vi "2021_day3_task2.vi"() -> ()   [LabVIEW 2021]
panel:
  out "life support rating":i32
  out "CO2 scrubber rating":i32
  out "oxygen generator rating":i32
  out "power consumption":u32
  out "Epsilon (DEC)":u32
  out "Gamma (DEC)":u32
  out "GAMA":bool[](array[boolean])
  out "EPSILON":bool[](array[boolean])
  out "size(s)":i32
  out "Array 2":i32[](array[numeric])
  out "Array":i32[][](array[numeric])
  out "array 2":string[](array[string])
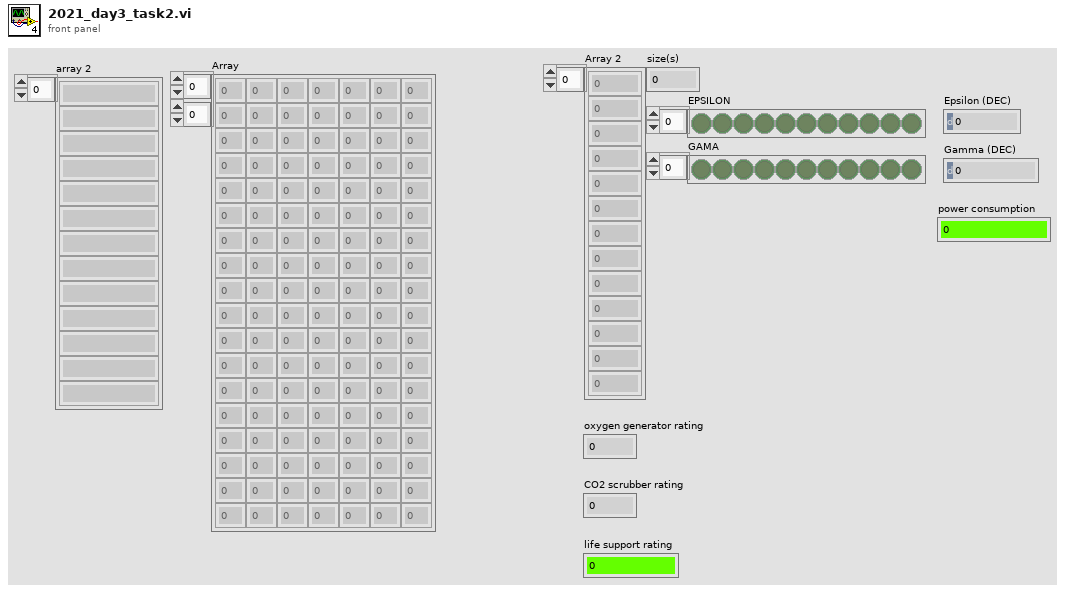
[diagram p1: front panel]
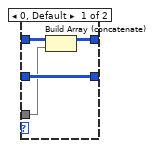
[diagram p2: hidden frame]
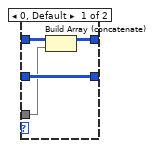
[diagram p3: hidden frame]
diagram:
  (unwired) "00100\n11110\n10110\n10111\n10101\n01111\n00111\n11100\n10000\n11001\n00010\n01010"
  n1 = Spreadsheet String To Array(delimiter (Tab)="\n", format string="%s", spreadsheet string="000111111001\n111011110110\n101111111000\n111100100110\n001111011000\n011100010110\n000101001001\n100001100101\n000011111100\n110000101000\n011110110101\n011000111100\n011000001011\n010111101101\n011111100010\n100110001111\n100111100100\n111110010100\n101001001110\n110101111110\n110110100000\n001010001110\n101100001100\n111001011000\n100101111111\n001001010100\n100111011000\n100101100000\n010001010101\n000111001100\n001100011110\n101100010101\n111011000011\n010000001110\n110000000110\n001010110000\n100011001111\n110100111101\n111111010100\n000101110111\n011110101111\n100110000110\n010011000000\n000110010000\n101101101011\n011101100011\n01...", array type (2D Dbl)=string[] []) -> (array=w28:string[])
  "array 2" <- w28
  n2 = for {
    tunnel: w28 -> [w36] mode=indexing
    tunnel: [w34] -> w7 mode=indexing
    n3 = String Length(string=w36) -> (length=w37:i32)
    n4 = for {
      N: w37 -> [_]
      shift-right: [w40] -> _
      shift-left: w36 -> [w40]
      tunnel: [w38] -> w35 mode=indexing
      i -> [w39]
      n5 = String Subset(string=w40, offset (0)=w39, length (rest)=1 ("length (rest)")) -> (substring=w38:string)
    }
    n6 = Decimal String To Number(string=w35) -> (number=w34:i32[])  [unwired: 2 in, 1 out]
  }
  "Array" <- w7
  n7 = Array Size(array=w28) -> (size(s)=w27:i32)
  "size(s)" <- w27
  n8 = Divide(x=w27, y=2) -> (x/y=w26:dbl)
  n9 = while {
    shift-right: [w44] -> w8
    shift-left: w7 -> [w50]
    i -> [w43]
    stop <- w42 stop-if-true
    w53 = i32[][] [] ("transposed array")
    # "1"
    # "0"
    n10 = Index Array(array=w50, index (col)=w43) -> (element=w54:i32[])  [unwired: 1 in]
    n11 = for {
      shift-right: [w61] -> w46
      shift-left: w53 -> [w60]
      shift-right: [w59] -> w45
      shift-left: w53 -> [w58]
      tunnel: w54 -> [w62] mode=indexing
      tunnel: w50 -> [w57]
      i -> [w55]
      n12 = Index Array(array=w57, index (row)=w55) -> (element=w56:i32[])  [unwired: 1 in]
      n13 = case shown="1" w62 {
        tunnel: [w64 w70] -> w61
        tunnel: w60 -> [w66 w70]
        tunnel: [w65 w68] -> w59
        tunnel: w58 -> [w65 w69]
        tunnel: w56 -> [w63 w67]
        frame 0, Default {
          n14 = Build Array (concatenate)(w66, w63) -> (w64:i32[][])
        }
        frame 1 {
          n15 = Build Array (concatenate)(w69, w67) -> (w68:i32[][])
        }
      }
    }
    n16 = Matrix Size(0:w46) -> (1:w49:i32)  [unwired: 1 out]
    n17 = Matrix Size(0:w45) -> (1:w48:i32)  [unwired: 1 out]
    n18 = Less Or Equal?(x=w49, y=w48) -> (x <= y?=w47:bool)
    n19 = Select(t=w46, s=w47, f=w45) -> (s? t:f=w44:i32[][])
    n20 = Matrix Size(0:w44) -> (1:w52:i32)  [unwired: 1 out]
    n21 = Equal?(x=w52, y=1) -> (x = y?=w42:bool)
  }
  n22 = while {
    shift-right: [w71] -> w17
    shift-left: w7 -> [w79]
    i -> [w78]
    stop <- w72 stop-if-true
    w82 = i32[][] [] ("transposed array")
    # "1"
    # "0"
    n23 = Index Array(array=w79, index (col)=w78) -> (element=w83:i32[])  [unwired: 1 in]
    n24 = for {
      shift-right: [w90] -> w74
      shift-left: w82 -> [w89]
      shift-right: [w88] -> w73
      shift-left: w82 -> [w87]
      tunnel: w83 -> [w91] mode=indexing
      tunnel: w79 -> [w86]
      i -> [w84]
      n25 = Index Array(array=w86, index (row)=w84) -> (element=w85:i32[])  [unwired: 1 in]
      n26 = case shown="1" w91 {
        tunnel: [w93 w99] -> w90
        tunnel: w89 -> [w95 w99]
        tunnel: [w94 w97] -> w88
        tunnel: w87 -> [w94 w98]
        tunnel: w85 -> [w92 w96]
        frame 0, Default {
          n27 = Build Array (concatenate)(w95, w92) -> (w93:i32[][])
        }
        frame 1 {
          n28 = Build Array (concatenate)(w98, w96) -> (w97:i32[][])
        }
      }
    }
    n29 = Matrix Size(0:w74) -> (1:w77:i32)  [unwired: 1 out]
    n30 = Matrix Size(0:w73) -> (1:w76:i32)  [unwired: 1 out]
    n31 = Greater?(x=w77, y=w76) -> (0:w75:bool)
    n32 = Select(t=w74, s=w75, f=w73) -> (s? t:f=w71:i32[][])
    n33 = Matrix Size(0:w71) -> (1:w81:i32)  [unwired: 1 out]
    n34 = Equal?(x=w81, y=1) -> (x = y?=w72:bool)
  }
  n35 = Transpose 2D Array(2D array=w7) -> (transposed array=w30:i32[][])
  n36 = for {
    tunnel: w30 -> [w103] mode=indexing
    tunnel: [w102] -> w29 mode=indexing
    tunnel: w26 -> [w101]
    tunnel: [w100] -> w24 mode=indexing
    n37 = Add Array Elements(numeric array=w103) -> (sum=w102:i32)
    n38 = Greater?(x=w101, y=w102) -> (0:w100:bool)
  }
  "Array 2" <- w29
  "EPSILON" <- w24
  n39 = Not(x=w24) -> (.not. x?=w23:bool[])
  "GAMA" <- w23
  n40 = Reverse 1D Array(array=w24) -> (reversed array=w21:bool[])
  n41 = Reverse 1D Array(array=w23) -> (reversed array=w22:bool[])
  n42 = Boolean Array To Number(Boolean array=w22) -> (number=w20:u32)
  "Gamma (DEC)" <- w20
  n43 = Boolean Array To Number(Boolean array=w21) -> (number=w19:u32)
  "Epsilon (DEC)" <- w19
  n44 = Multiply(x=w20, y=w19) -> (x*y=→"power consumption":u32)
  n45 = Index Array(array=w8, index (row)=0) -> (element=w12:i32[])  [unwired: 1 in]
  n46 = Index Array(array=w17, index (row)=0) -> (element=w13:i32[])  [unwired: 1 in]
  n47 = To Unsigned Byte Integer(number=w13) -> (unsigned 8bit integer=w3:u8[])
  n48 = To Unsigned Byte Integer(number=w12) -> (unsigned 8bit integer=w2:u8[])
  n49 = for {
    tunnel: w2 -> [w105] mode=indexing
    tunnel: [w104] -> w10 mode=concatenating
    n50 = Number To Decimal String(number=w105) -> (decimal integer string=w104:string)  [unwired: 1 in]
  }
  n51 = for {
    tunnel: w3 -> [w107] mode=indexing
    tunnel: [w106] -> w15 mode=concatenating
    n52 = Number To Decimal String(number=w107) -> (decimal integer string=w106:string)  [unwired: 1 in]
  }
  n53 = Scan From String(format string="%b", input string=w10) -> (output 1=w5:i32)  [unwired: 3 in, 3 out]
  "CO2 scrubber rating" <- w5
  n54 = Scan From String(format string="%b", input string=w15) -> (output 1=w6:i32)  [unwired: 3 in, 3 out]
  "oxygen generator rating" <- w6
  n55 = Multiply(x=w6, y=w5) -> (x*y=→"life support rating":i32)
